vi "SpecificVI - End Modal SubVI.vi"(0 "VI Originally Open":bool, 1 "error out":errorcluster, 2 "Modal ID":i32, 3 "This VI":refnum<vi>, 4 "Sequence Context Out":refnum<k7>) -> ()   [LabVIEW 2009]
uses:
  <vilib>/addons/TestStand/_TSUtility.llb/TestStand - End Modal Dialog (Sequence Context).vi
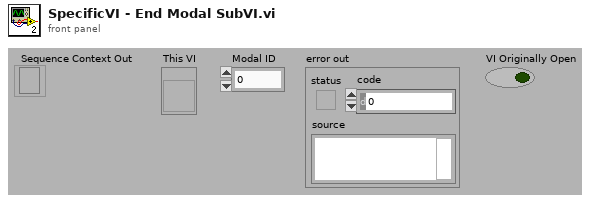
[diagram p1: front panel]
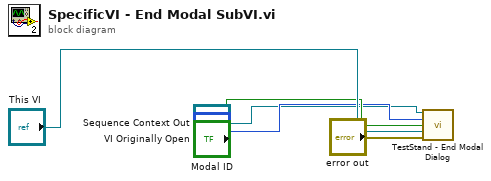
[diagram p0: block diagram]
diagram:
  n1 = call-poly <vilib>:"TestStand - End Modal Dialog.vi"("Sequence Context In"="Sequence Context Out", "Modal ID"="Modal ID", "VI Originally Open"="VI Originally Open", "VI to make non-Modal (Current VI)"="This VI", "error in (no error)"="error out") -> ()  [unwired: 10 in, 1 out]
